vi "FastMap - Eliminated.vi"(8 "Column":i32, 9 "Row":i32, 10 "Last Position":T1, 11 "fast map in":refnum<data-value>) -> (3 "fast map out":refnum<data-value>)   [LabVIEW 2020, in "DS Square.lvlib"]
uses:
  DS Square.lvlib
  Fast Map.ctl
  Square State Fast.ctl
  Common/Position.ctl
  Common/Common.lvlib
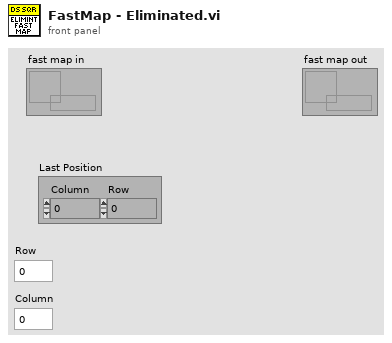
[diagram p1: front panel]
types:
  T1 = typedef "Common.lvlib/Position.ctl" = cluster{"Column":i32, "Row":i32}
  T2 = typedef "DS Square.lvlib/Square State Fast.ctl" = enum8{"Unknown", "Empty", "Occupied - Active", "Occupied - Cool Down", "Attacked", "Enemy", "Enemy Wall"}
  T3 = typedef "DS Square.lvlib/Fast Map.ctl" = cluster{"state":T2[][], "updated":i32[][]}
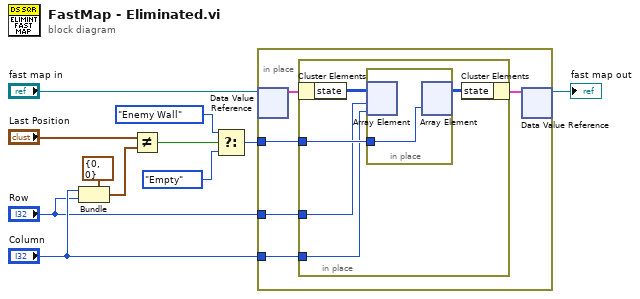
[diagram p0: block diagram]
diagram:
  n1 = Bundle(cluster=T1 {"Column"=0, "Row"=0} ("Position in"), "Column"="Column", "Row"="Row") -> (w7:T1)
  n2 = Not Equal?(x="Last Position", y=w7) -> (x != y?=w6:bool)
  n3 = Select(t=Square_State_Fast."Enemy Wall" ("square state"), s=w6, f=Square_State_Fast."Empty" ("square state")) -> (s? t:f=w3:T2)
  n4 = in-place {
    in-place-border: w3 -> [w15]
    in-place-border: "Column" -> [w14]
    in-place-border: "Row" -> [w13]
    n5 = in-place-dvr #1("fast map in") -> (w16:T3)  [unwired: 1 out]
    n6 = in-place {
      in-place-border: w15 -> [w20]
      in-place-border: w14 -> [w19]
      in-place-border: w13 -> [w18]
      n7 = in-place-cluster #2(w16) -> ("state"=w21:T2[][])
      n8 = in-place {
        in-place-border: w20 -> [w22]
        n9 = in-place-array #3(w21, w18, w19) -> ()  [unwired: 1 out]
        n10 = in-place-array #3(w22) -> (w17:T2[][])  [unwired: 2 out]
      }
      n11 = in-place-cluster #2("state"=w17) -> (w12:T3)
    }
    n12 = in-place-dvr #1(w12) -> (→"fast map out":refnum<data-value>)  [unwired: 1 out]
  }
